vi "U6 PWM and Quadrature Loop.vi"(9 "Timer0 Duty Cycle [%]":dbl=50.0 format="%.1f", 10 "16-bit PWM Frequency [Hz]":dbl=40.0 format="%.2f") -> (2 "Actual 16-bit Frequency":dbl format="%.1f")   [LabVIEW 2021]
panel:
  out "Timer2":i32
  in  "Timer/Counter Pin Offset":u8
  out "Update":bool
  out "Timer Value Array":u16[](array[numeric])
  in  "Timer1 Duty Cycle [%]":dbl=50.0 format="%.1f"
  in  "stop":bool
  out "Actual 8-bit Frequency":dbl format="%.1f"
  in  "FirstFound":bool=TRUE
  in  "Address":string="1"
  out "TimerClockDivisor":u8
  out "Error Message":string
  # "Demonstrates 1 channel of PWM16, 1 channel of PWM8, and 2 other timers configured\nas a quadrature pair.\nUses the 48 MHz divisor capable clock, and chooses a timer clock divisor to get\nas close as possible to the desired 16-bit PWM frequency.  Since a divisor capable\nclock is used, Counter0 is not available.  Since all timers use the same clock, the\nfrequency of the 8-bit PWM is fixed at 256 times the frequency of the 16-bit PWM.\nIf pin offset is 0, we get:\n\nFIO0 = PWM16, FIO1 = PWM16, FIO2/3 = Quadrature"
  # "Range is 2.86 to 732.42 Hz"
  # "This example allows the duty cycles to\nbe changed while the VI is running, but\nnot frequency."
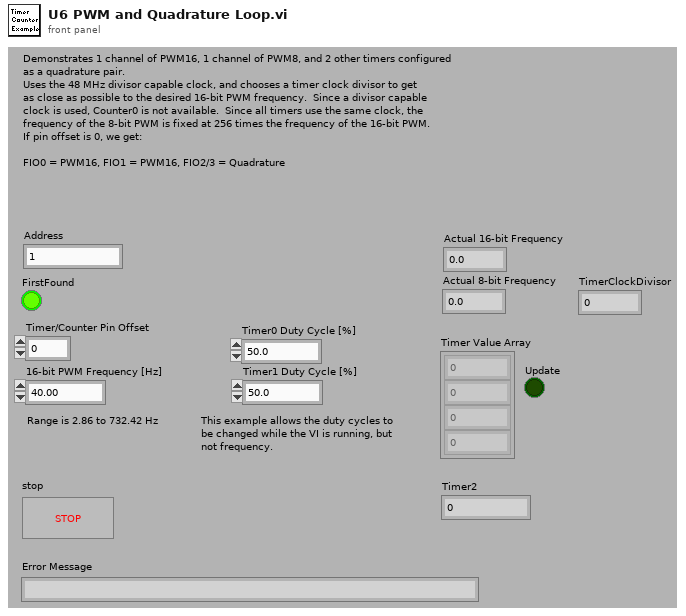
[diagram p1: front panel]
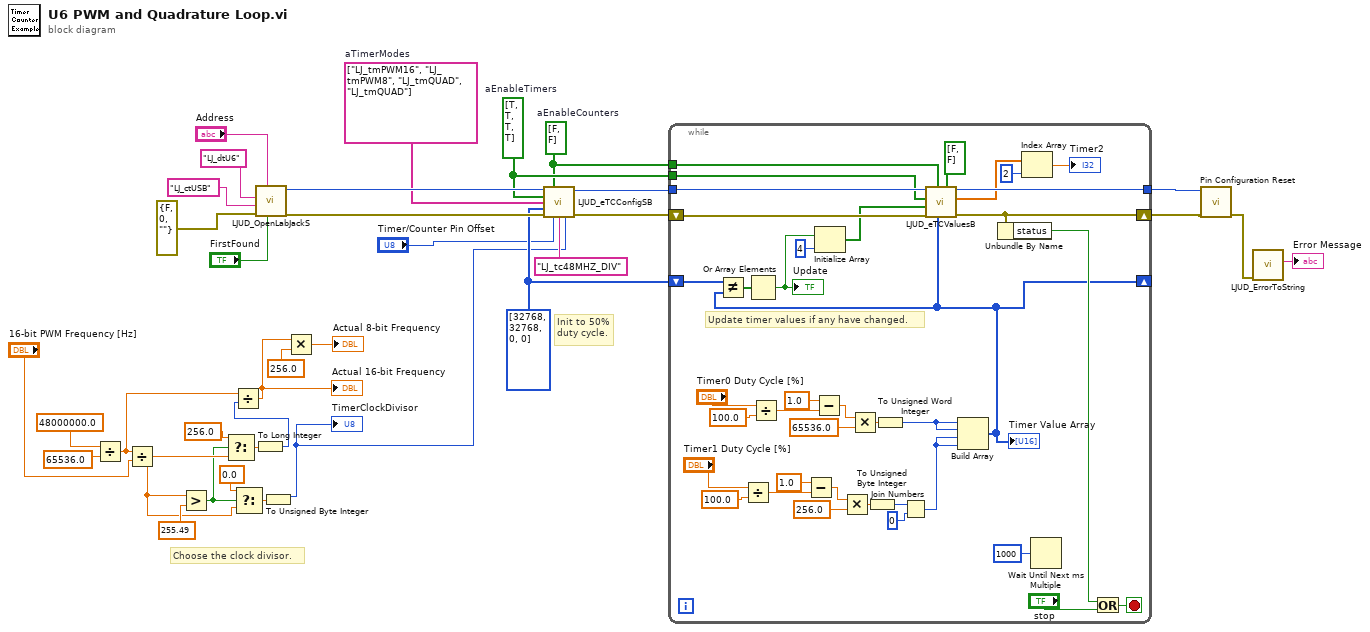
[diagram p0: block diagram]
diagram:
  w1 = bool[] [FALSE, FALSE]  # aEnableCounters
  w3 = bool[] [TRUE, TRUE, TRUE, TRUE]  # aEnableTimers
  w8 = string[] ["LJ_tmPWM16", "LJ_tmPWM8", "LJ_tmQUAD", "LJ_tmQUAD"]  # aTimerModes
  w7 = u16[] [32768, 32768, 0, 0] ("TimerValues")
  # "Choose the clock divisor."
  # "Init to 50%\nduty cycle."
  n1 = Divide(x=48000000.0, y=65536.0) -> (x/y=w23:dbl)
  n2 = Divide(x=w23, y="16-bit PWM Frequency [Hz]") -> (x/y=w27:dbl)
  n3 = Greater?(x=w27, y=255.49) -> (0:w26:bool)
  n4 = Select(t=256.0, s=w26, f=w27) -> (s? t:f=w29:dbl)
  n5 = Select(t=0.0, s=w26, f=w27) -> (s? t:f=w32:dbl)
  n6 = To Long Integer(number=w29) -> (32bit integer=w25:i32)
  n7 = Divide(x=w23, y=w25) -> (x/y=w22:dbl)
  "Actual 16-bit Frequency" <- w22
  n8 = call "LJUD_OpenLabJackS.vi"("FirstFound"="FirstFound", "Address"="Address", "error in"=errorcluster {"status"=FALSE, "code"=0, "source"=""}, "ConnectionType"="LJ_ctUSB", "DeviceType"="LJ_dtU6") -> ("error out"=w9:errorcluster, "Handle"=w10:i32)  [unwired: 4 in, 1 out]
  n9 = To Unsigned Byte Integer(number=w32) -> (unsigned 8bit integer=w4:u8)
  "TimerClockDivisor" <- w4
  n10 = Multiply(x=w22, y=256.0) -> (x*y=→"Actual 8-bit Frequency":dbl)
  n11 = call "LJUD_eTCConfigSB.vi"("Handle In"=w10, "aEnableCounters"=w1, "aEnableTimers"=w3, "aTimerModes"=w8, "aTimerValues"=w7, "error in"=w9, "TCPinOffset"="Timer/Counter Pin Offset", "TimerClockBase"="LJ_tc48MHZ_DIV" ("Timer Clock Base"), "TimerClockDivisor"=w4) -> ("Handle Out"=w11:i32, "error out"=w12:errorcluster)  [unwired: 5 in]
  n12 = while {
    tunnel: w3 -> [w45]
    tunnel: [w50] -> w19
    shift-left: w7 -> [w57]
    shift-right: [w43] -> _
    tunnel: w11 -> [w47]
    shift-left: w12 -> [w48]
    shift-right: [w49] -> w18
    tunnel: w1 -> [w40]
    stop <- w58 stop-if-true
    # "Update timer values if any have changed."
    n13 = Divide(x="Timer1 Duty Cycle [%]", y=100.0) -> (x/y=w71:dbl)
    n14 = Divide(x="Timer0 Duty Cycle [%]", y=100.0) -> (x/y=w63:dbl)
    n15 = Subtract(x=1.0, y=w71) -> (x-y=w69:dbl)
    n16 = Subtract(x=1.0, y=w63) -> (x-y=w61:dbl)
    n17 = Multiply(x=w69, y=256.0) -> (x*y=w66:dbl)
    n18 = Multiply(x=w61, y=65536.0) -> (x*y=w60:dbl)
    n19 = To Unsigned Byte Integer(number=w66) -> (unsigned 8bit integer=w68:u8)
    n20 = To Unsigned Word Integer(number=w60) -> (unsigned 16bit integer=w41:u16)
    n21 = Join Numbers(hi=w68, lo=u8 0) -> ((hi.lo)=w42:u16)
    n22 = Build Array(w41, w41, w42, w42) -> (w43:u16[])
    "Timer Value Array" <- w43
    n23 = Not Equal?(x=w57, y=w43) -> (x != y?=w56:bool[])
    n24 = Or Array Elements(Boolean array=w56) -> (logical OR=w55:bool)
    "Update" <- w55
    n25 = Initialize Array(w55, 4 ("Dimension Size")) -> (w46:bool[])
    n26 = call "LJUD_eTCValuesB.vi"("aResetCounters"=bool[] [FALSE, FALSE] ("aEnableCounters"), "aTimerValues Write"=w43, "aReadCounters"=w40, "error in"=w48, "aUpdateResetTimers"=w46, "aReadTimers"=w45, "Handle In"=w47) -> ("error out"=w49:errorcluster, "aTimerValues Read"=w36:dbl[], "Handle Out"=w50:i32)  [unwired: 1 in, 1 out]
    n27 = Unbundle By Name(w49) -> ("status"=w54:bool)
    n28 = Index Array(array=w36, index=2) -> (element=→"Timer2":dbl)
    n29 = Wait Until Next ms Multiple(millisecond multiple=u32 1000) -> ()  [unwired: 1 out]
    n30 = Or(x=w54, y="stop") -> (x .or. y?=w58:bool)
  }
  n31 = call "Pin Configuration Reset.vi"("error in"=w18, "Handle In"=w19) -> ("error out"=w17:errorcluster)  [unwired: 8 in, 1 out]
  n32 = call "LJUD_ErrorToString.vi"("error in"=w17) -> ("String"=→"Error Message":string)  [unwired: 10 in]
